vi "Create Sysdef and Add New Custom Device w. 1000 chans.vi"() -> ()   [LabVIEW 2010]
uses:
  NationalInstruments.VeriStand.SystemDefinitionAPI
  Read RefMem PtByPt System Definition API.lvlibp/API/Channel Config.ctl
  Read RefMem PtByPt System Definition API.lvlibp
panel:
  in  "# to create":i32=1000
  in  "VISA Name":string="RM"
  in  "Device Name":string="My RefMem Reader"
  in  "Sysdef File to create":path
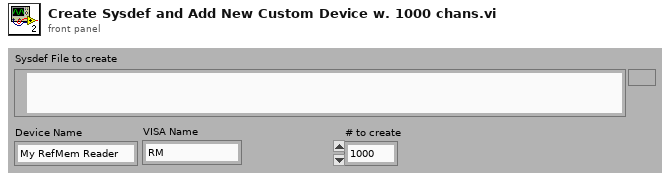
[diagram p1: front panel]
types:
  T1 = typedef "SysDefRefs.ctl" = cluster{"SysDef Ref":refnum<k24>, "Root Node":refnum<k24>, "Targets Section":refnum<k24>, "Target List":refnum<k24>[], "CD Section":refnum<k24>, "CustomDeviceList":refnum<k24>[]}
  T2 = typedef "Read RefMem PtByPt System Definition API.lvlibp/Channel Config.ctl" = cluster{"Units":string, "Default Value":dbl, "Address":u32, "Description":string}
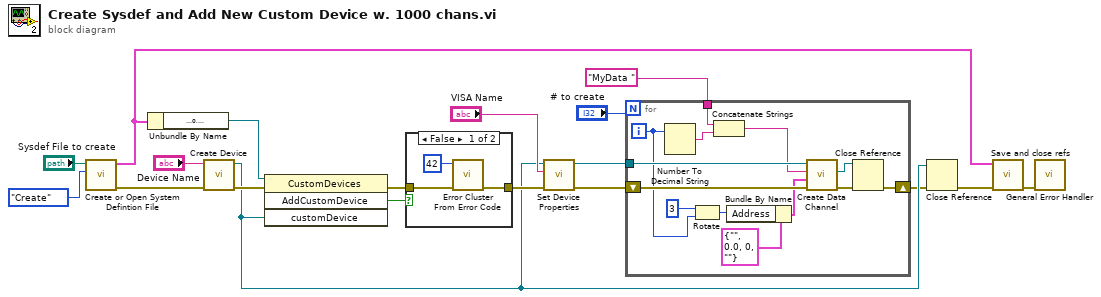
[diagram p0: block diagram]
diagram:
  n1 = call "Create or Open System Defintion File.vi"("File Action"=enum16{"Open", "Create"}."Create", "Sysdef File"="Sysdef File to create") -> ("error out"=w10:errorcluster, "SysDef Refs"=w15:T1)  [unwired: 8 in]
  n2 = Unbundle By Name(w15) -> ("CD Section"=w14:refnum<k24>)
  n3 = call "Create Device.vi"("error in (no error)"=w10, "Name"="Device Name") -> ("error out"=w4:errorcluster, "Custom Device"=w2:refnum<k24>)  [unwired: 8 in]
  n4 = invoke class="CustomDevices" method="AddCustomDevice"(reference=w14, error in=w4, "customDevice"=w2) -> (error out=w17:errorcluster, "AddCustomDevice"=w16:bool)  [unwired: 1 in, 2 out]
  n5 = case shown="False" w16 {
    tunnel: [w21 w23] -> w3
    tunnel: w17 -> [w20 w23]
    frame False {
      n6 = call <vilib>:"Error Cluster From Error Code.vi"("error in (no error)"=w20, "error code (0)"=42) -> ("error out"=w21:errorcluster)  [unwired: 7 in]
    }
    frame True {
    }
  }
  n7 = call "Set Device Properties.vi"("error in (no error)"=w3, "VISA Name"="VISA Name", "Custom Device"=w2) -> ("error out"=w8:errorcluster, "Custom Device Duplicate"=w7:refnum<k24>)  [unwired: 7 in]
  n8 = for {
    N: "# to create" -> [_]
    shift-right: [w24] -> w1
    shift-left: w8 -> [w36]
    tunnel: w7 -> [w35]
    tunnel: "MyData " ("Data Channel Name") -> [w34]
    i -> [w27]
    n9 = Number To Decimal String(number=w27) -> (decimal integer string=w33:string)  [unwired: 1 in]
    n10 = Rotate(1:w27, 2:i8 3 ("y")) -> (0:w28:i32)
    n11 = Concatenate Strings(w34, w33) -> (w32:string)
    n12 = Bundle By Name(cluster=T2 {"Units"="", "Default Value"=0.0, "Address"=0, "Description"=""} ("Channel"), "Address"=w28) -> (w30:T2)
    n13 = call "Create Data Channel.vi"("error in (no error)"=w36, "Channel"=w30, "Name"=w32, "Parent Section"=w35) -> ("error out"=w26:errorcluster, "New Data Channel"=w25:refnum<k24>)  [unwired: 4 in, 2 out]
    n14 = Close Reference(reference=w25, error in (no error)=w26) -> (error out=w24:errorcluster)
  }
  n15 = Close Reference(reference=w2, error in (no error)=w1) -> (error out=w13:errorcluster)
  n16 = call "Save and close refs.vi"("error in (no error)"=w13, "SysDef Refs in"=w15) -> ("error out"=w18:errorcluster)  [unwired: 9 in]
  n17 = call <vilib>:"General Error Handler.vi"("error in (no error)"=w18) -> ()  [unwired: 10 in, 5 out]
